vi "SetRegisters.vi"(7 "Lenght":i32, 8 "error in (no error)":errorcluster, 9 "Register Data":u8[](array[numeric]), 10 "Register Addres":u8[](array[numeric]), 11 "BME680 in":refnum<class "BME680.lvclass">) -> (0 "error out":errorcluster, 3 "BME680 out":refnum<class "BME680.lvclass">)   [LabVIEW 2022 SP3, in "BME680.lvlib" / "BME680.lvclass"]
uses:
  BME680.lvclass
  BME680.lvclass/BME680.ctl
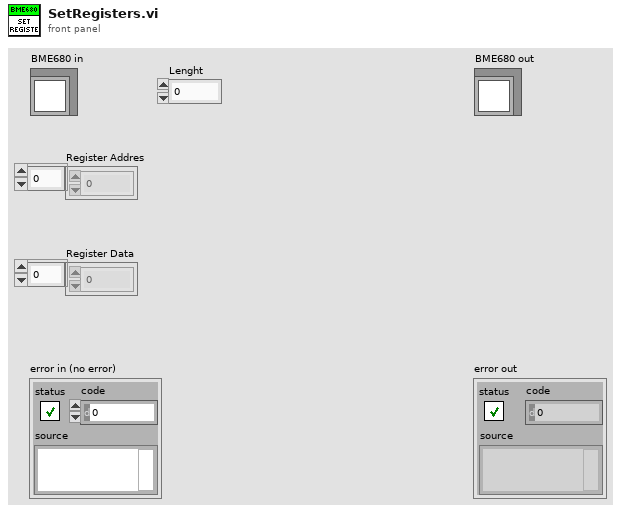
[diagram p1: front panel]
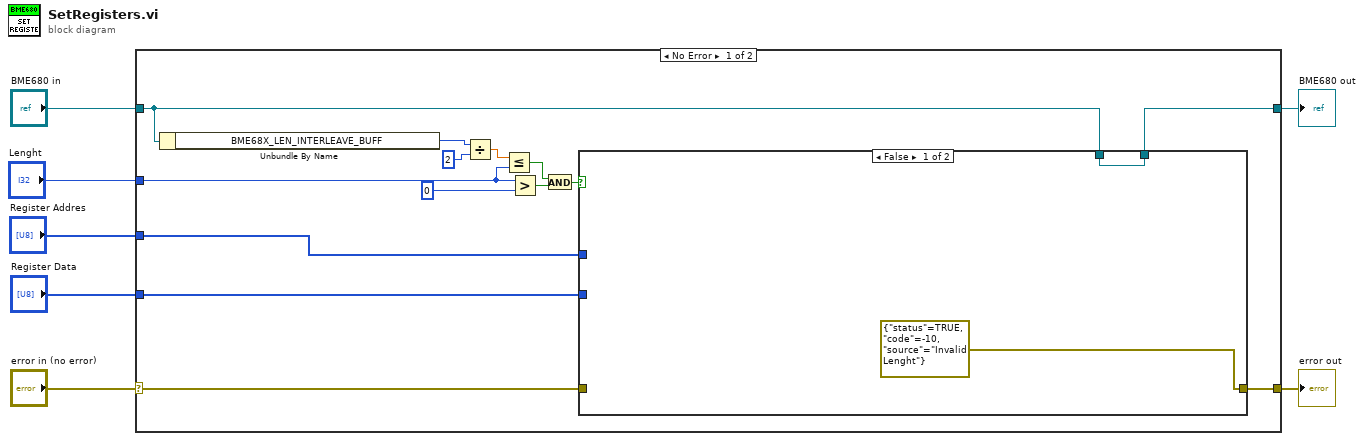
[diagram p0: block diagram]
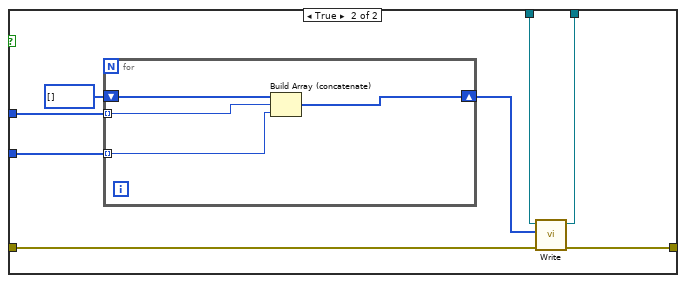
[diagram p2: hidden frame]
diagram:
  n1 = case shown="No Error" "error in (no error)" {
    selector: "error in (no error)" -> [w17 w37]
    tunnel: [w16 w37] -> w6
    tunnel: [w18 w36] -> w4
    tunnel: "BME680 in" -> [w19 w36]
    tunnel: "Register Addres" -> [w21 _]
    tunnel: "Register Data" -> [w20 _]
    tunnel: "Lenght" -> [w12 _]
    frame No Error {
      n2 = Unbundle By Name(w19) -> ("BME68X_LEN_INTERLEAVE_BUFF"=w9:u8)
      n3 = Divide(x=w9, y=u8 2) -> (x/y=w10:dbl)
      n4 = Less Or Equal?(x=w10, y=w12) -> (x <= y?=w13:bool)
      n5 = Greater?(x=w12, y=0) -> (0:w14:bool)
      n6 = And(x=w13, y=w14) -> (x .and. y?=w11:bool)
      n7 = case shown="False" w11 {
        tunnel: w21 -> [_ w31]
        tunnel: w20 -> [_ w30]
        tunnel: w19 -> [w23 w27]
        tunnel: [w23 w26] -> w18
        tunnel: w17 -> [_ w25]
        tunnel: [errorcluster {"status"=TRUE, "code"=-10, "source"="Invalid Lenght"} ("error out") w24] -> w16
        frame False {
        }
        frame True {
          n8 = for {
            tunnel: w31 -> [w35] mode=indexing
            tunnel: w30 -> [w34] mode=indexing
            shift-right: [w33] -> w28
            shift-left: u8[] [] -> [w32]
            n9 = Build Array (concatenate)(w32, w35, w34) -> (w33:u8[])
          }
          n10 = call "Write.vi"("error in (no error)"=w25, "Data"=w28, "BME680 in"=w27) -> ("error out"=w24:errorcluster, "BME680 out"=w26:refnum<class "BME680.lvclass">)  [unwired: 7 in]
        }
      }
    }
    frame Error {
    }
  }
  "error out" <- w6
  "BME680 out" <- w4
